vi "BRig_dataCurrent_init.vi"() -> (3 "output_dataCurrent":u16[](array[numeric]))   [LabVIEW 2014]
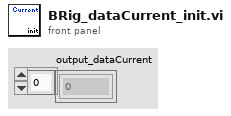
[diagram p1: front panel]
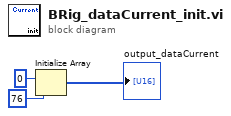
[diagram p0: block diagram]
diagram:
  n1 = Initialize Array(u16 0 ("element"), 76 ("dimension size")) -> (→"output_dataCurrent":u16[])
